vi "Draw.vi"(8 "error in (no error)":errorcluster, 11 "Circle in":refnum<class "Circle.lvclass">) -> (0 "error out":errorcluster, 2 "Shape":picture, 3 "Circle out":refnum<class "Circle.lvclass">)   [LabVIEW 2019, in "Circle.lvclass"]
uses:
  Circle.lvclass
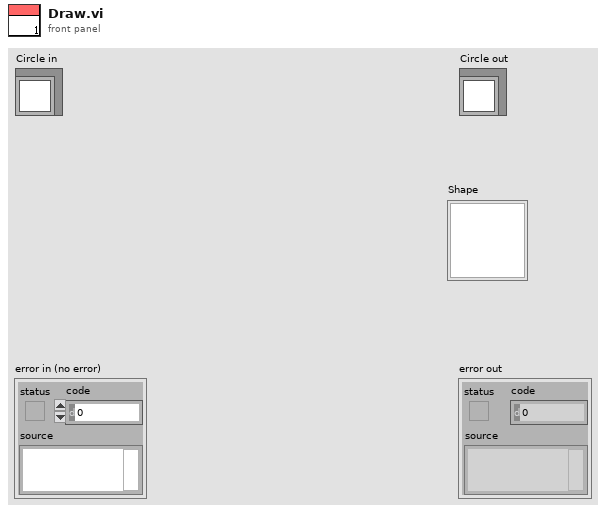
[diagram p1: front panel]
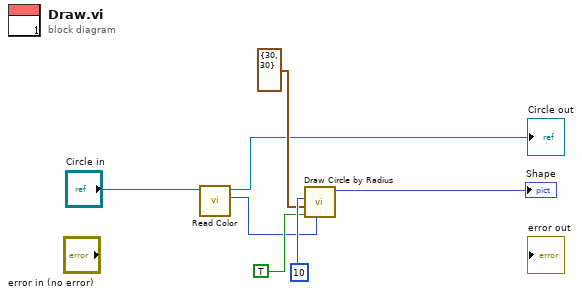
[diagram p0: block diagram]
diagram:
  n1 = call-dynamic "Read Color.vi"("Shape in"="Circle in") -> ("Color"=w3:u32, "Shape out"=→"Circle out":refnum<class "Circle.lvclass">)  [unwired: 8 in, 1 out]
  n2 = call <vilib>:"Draw Circle by Radius.vi"("color(black)"=w3, "fill?(F)"=TRUE, "pixel center"=cluster{"horizontal":i16, "vertical":i16} {"horizontal"=30, "vertical"=30}, "radius"=i16 10) -> ("new picture"=→"Shape":picture)  [unwired: 7 in]
